vi "Get Keys to Read.vi"(8 "error in (no error)":errorcluster, 9 "Debug Build?":bool, 10 "Section Name":string, 11 "Config File":T1) -> (0 "error out":errorcluster, 2 "Keys to Read":string[][](array[string]), 3 "Config File":T1)   [LabVIEW 2019, in "PPL INI Parsing.lvlib"]
doc: "Creates a list of the keys specified in the Section specified by <b>Section Name</b>, or Name.{Release,Debug} where Release and Debug are chosen by the boolean control, <b>Debug Build?</b>."
uses:
  PPL INI Parsing.lvlib
  <vilib>/Utility/config.llb/Config Data RefNum.ctl
  <vilib>/Utility/config.llb/NI_LVConfig.lvlib
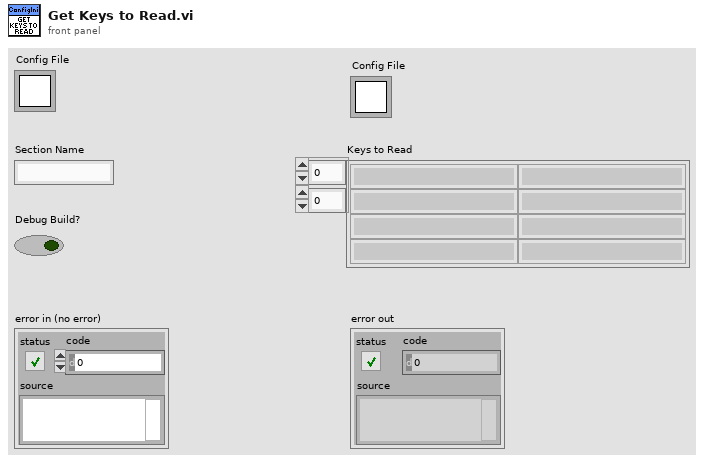
[diagram p1: front panel]
types:
  T1 = typedef "NI_LVConfig.lvlib/Config Data RefNum.ctl" = refnum<k1>
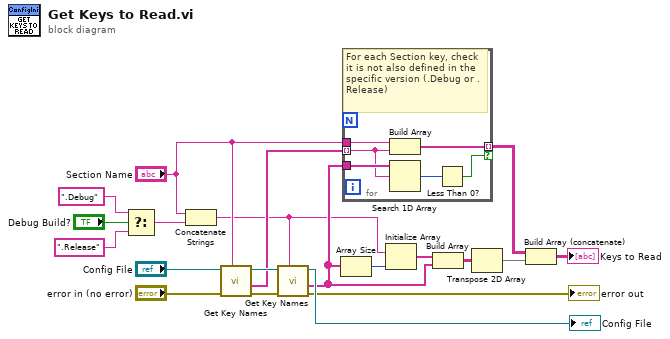
[diagram p0: block diagram]
diagram:
  n1 = Select(t=".Debug", s="Debug Build?", f=".Release") -> (s? t:f=w17:string)
  n2 = Concatenate Strings("Section Name", w17) -> (w2:string)
  n3 = call <vilib>:"Get Key Names.vi"("section"="Section Name", "error in (no error)"="error in (no error)", "refnum"="Config File") -> ("error out"=w12:errorcluster, "key names"=w10:string[], "refnum out"=w16:T1)  [unwired: 5 in, 1 out]
  n4 = call <vilib>:"Get Key Names.vi"("section"=w2, "error in (no error)"=w12, "refnum"=w16) -> ("error out"=→"error out":errorcluster, "key names"=w5:string[], "refnum out"=→"Config File":T1)  [unwired: 5 in, 1 out]
  n5 = Array Size(array=w5) -> (size(s)=w4:i32)
  n6 = for {
    tunnel: w10 -> [w22] mode=indexing
    tunnel: w5 -> [w26]
    tunnel: [w21] -> w8 mode=indexing if=w24
    tunnel: "Section Name" -> [w23]
    # "For each Section key, check it is not also defined in the specific version (.Debug or .Release)"
    n7 = Build Array(w23, w22) -> (w21:string[])
    n8 = Search 1D Array(1D array=w26, element=w22) -> (index of element=w25:i32)  [unwired: 1 in]
    n9 = Less Than 0?(x=w25) -> (x < 0?=w24:bool)
  }
  n10 = Initialize Array(w2, w4) -> (w6:string[])
  n11 = Build Array(w6, w5) -> (w3:string[][])
  n12 = Transpose 2D Array(2D array=w3) -> (transposed array=w1:string[][])
  n13 = Build Array (concatenate)(w8, w1) -> (→"Keys to Read":string[][])
